vi "extra q palindrome using index array.vi"() -> ()   [LabVIEW 2025]
panel:
  out "is palindrome":bool
  in  "String":string
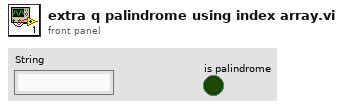
[diagram p1: front panel]
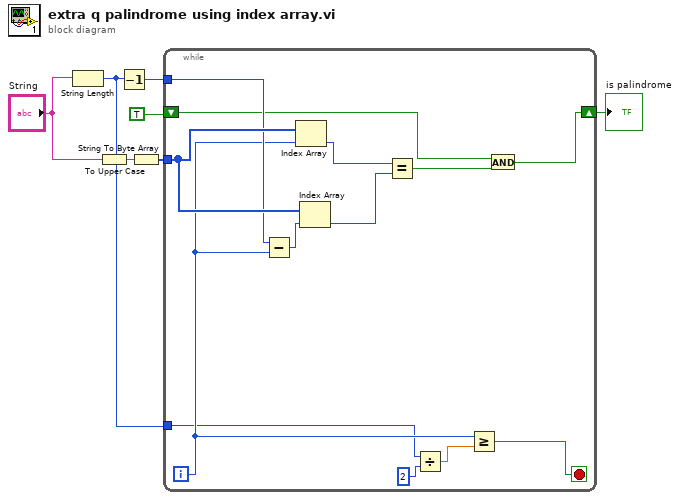
[diagram p0: block diagram]
diagram:
  n1 = String Length(string="String") -> (length=w3:i32)
  n2 = To Upper Case(1:"String") -> (0:w5:string)
  n3 = Decrement(x=w3) -> (x-1=w6:i32)
  n4 = String To Byte Array(string=w5) -> (unsigned byte array=w4:u8[])
  n5 = while {
    tunnel: w6 -> [w19]
    tunnel: w4 -> [w20]
    tunnel: w3 -> [w15]
    shift-right: [w8] -> w1
    shift-left: TRUE -> [w9]
    i -> [w17]
    stop <- w13 stop-if-true
    n6 = Subtract(x=w19, y=w17) -> (x-y=w18:i32)
    n7 = Index Array(array=w20, index=w17) -> (element=w12:u8)
    n8 = Index Array(array=w20, index=w18) -> (element=w11:u8)
    n9 = Equal?(x=w12, y=w11) -> (x = y?=w10:bool)
    n10 = Divide(x=w15, y=2) -> (x/y=w14:dbl)
    n11 = Greater Or Equal?(x=w17, y=w14) -> (x >= y?=w13:bool)
    n12 = And(x=w9, y=w10) -> (x .and. y?=w8:bool)
  }
  "is palindrome" <- w1
